vi "CT_PSOverVoltageCheck.vi"(0 "PS Array":T1[](array[typedef]) {"Feedback Voltage (kV)" format="%#_2f"; "Charge Voltage (kV)" format="%#_2f"; "Charge Current (A)" format="%#.2e"; "Capacitance per load" format="%#.2e"}) -> (1 "Overvoltage":bool, 2 "PS ID":i32)   [LabVIEW 2016]
uses:
  PScluster.ctl
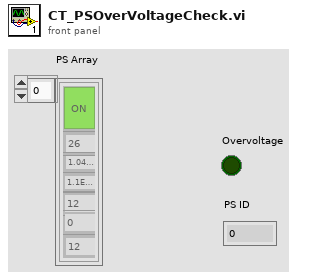
[diagram p1: front panel]
types:
  T1 = typedef "PScluster.ctl" = cluster{"On/Off Selector":bool, "Number of Loads":u32, "Capacitance per load":dbl, "Charge Current (A)":dbl, "Charge Voltage (kV)":dbl, "PWM calib":dbl, "Feedback Voltage (kV)":dbl}
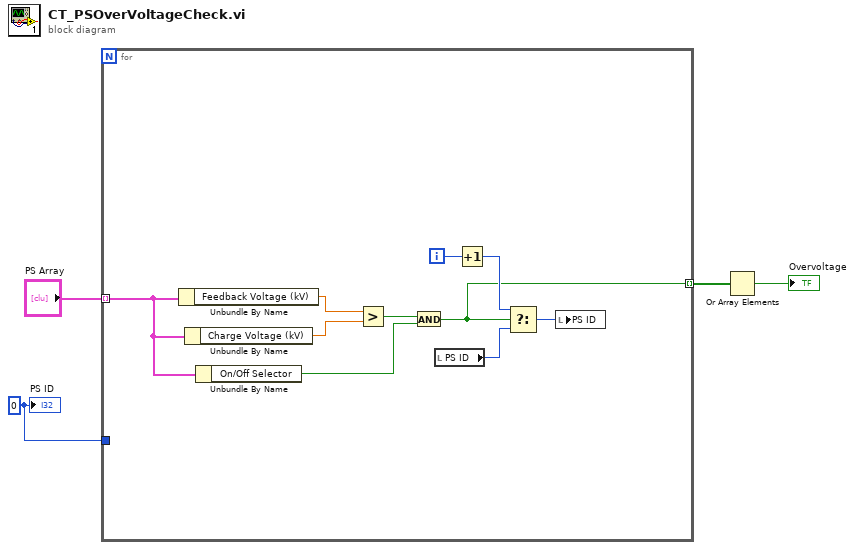
[diagram p0: block diagram]
diagram:
  w1 = 0 ("PS ID")
  n1 = for {
    tunnel: "PS Array" -> [w12] mode=indexing
    tunnel: [w7] -> w4 mode=indexing
    tunnel: w1 -> [_]
    i -> [w9]
    n2 = Unbundle By Name(w12) -> ("Feedback Voltage (kV)"=w14:dbl)
    n3 = Unbundle By Name(w12) -> ("Charge Voltage (kV)"=w13:dbl)
    n4 = Unbundle By Name(w12) -> ("On/Off Selector"=w10:bool)
    n5 = Greater?(x=w14, y=w13) -> (0:w11:bool)
    n6 = And(x=w11, y=w10) -> (x .and. y?=w7:bool)
    n7 = local read "PS ID"() -> (w5:i32)
    n8 = Increment(x=w9) -> (x+1=w8:i32)
    n9 = Select(t=w8, s=w7, f=w5) -> (s? t:f=w6:i32)
    n10 = local write "PS ID"(w6) -> ()
  }
  n11 = Or Array Elements(Boolean array=w4) -> (logical OR=→"Overvoltage":bool)
  "PS ID" <- w1
